vi "makeGraphLegend.vi"(7 "Front Panel Window:Minimum Size":T1, 10 "NewBnds":T2, 11 "XYGraph in":refnum<vi>) -> ()   [LabVIEW 2022 SP3]
uses:
  <vilib>/Utility/miscctls.llb/LVRectTypeDef.ctl
  <vilib>/Utility/miscctls.llb/LVPointTypeDef.ctl
  Anemometry/Anemometry Sub Vis/Data_plotting_vis/Results_plotter_Global.vi
panel:
  in  "Graph:Position:Left":i32=1
  in  "Graph:Position:Top":i32=26
  in  "baseLegendWidthChars":u32=33
  in  "origPlotAreaWidth":u32=510
  in  "origPlotAreaHeight":u32=256
  in  "avPixelsPerChar":dbl=6.0 format="%#_13g"
  in  "legendOffsetFromPlotArea":u32=117
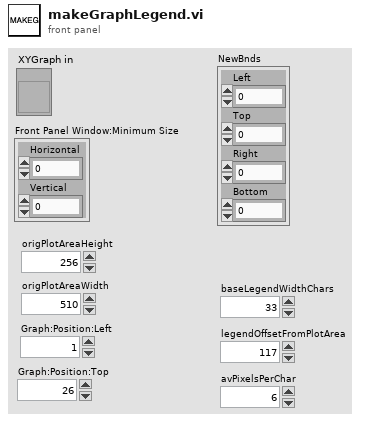
[diagram p1: front panel]
types:
  T1 = typedef "LVPointTypeDef.ctl" = cluster{"Horizontal":i16, "Vertical":i16}
  T2 = typedef "LVRectTypeDef.ctl" = cluster{"Left":i16, "Top":i16, "Right":i16, "Bottom":i16}
  T3 = cluster{"Plot Color":u32, "Plot Interpolation":u8, "Point Style":u8, "Line Style":u8, "Fill/Pt. Color":u32, "Line Width":u8, "Bar Plot Style":u8, "Fill To":i16}[]
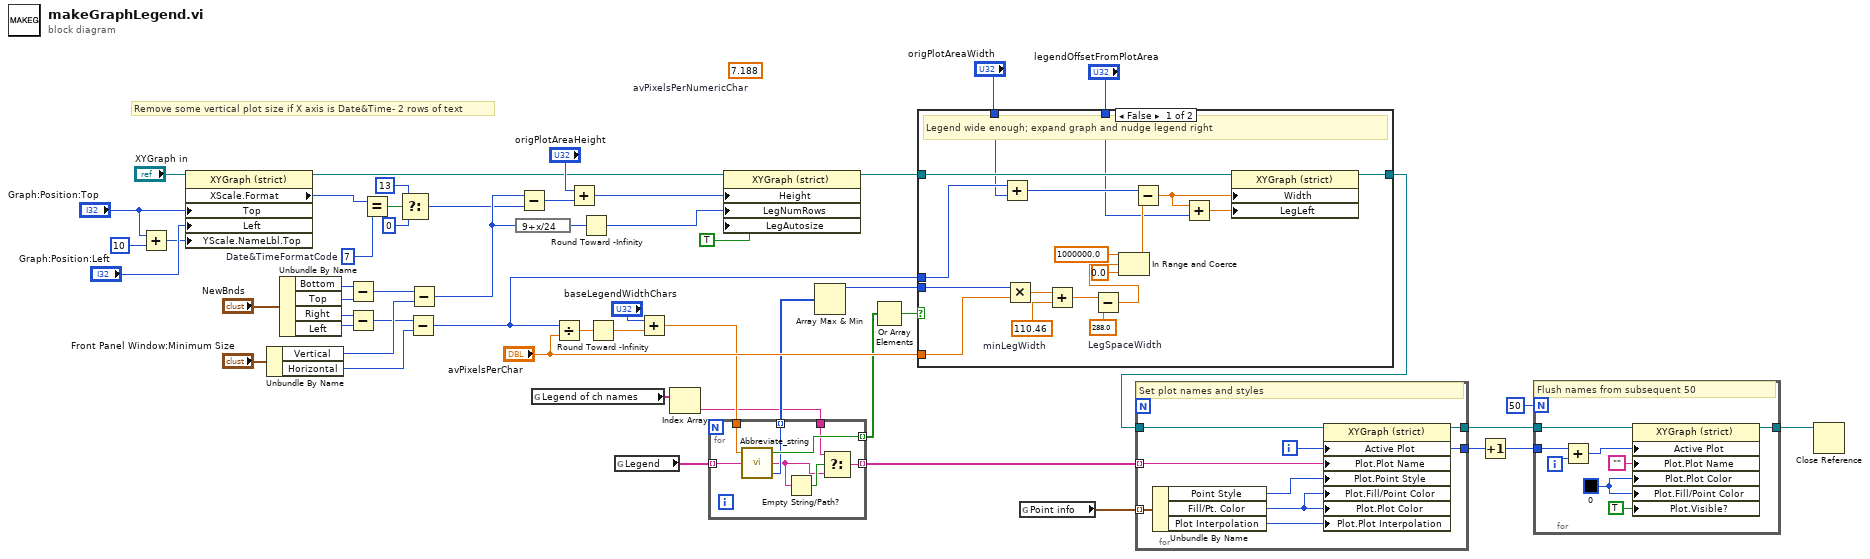
[diagram p0: block diagram]
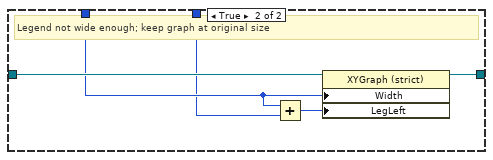
[diagram p2: hidden frame]
diagram:
  w12 = u8 7  # Date&TimeFormatCode
  (unwired) 7.188  # avPixelsPerNumericChar
  # "Remove some vertical plot size if X axis is Date&Time- 2 rows of text"
  n1 = Add(x="Graph:Position:Top", y=10) -> (x+y=w2:i32)
  n2 = property class="XYGraph (strict)"(reference="XYGraph in", "Top"="Graph:Position:Top", "Left"="Graph:Position:Left", "YScale.NameLbl.Top"=w2) -> (reference out=w14:refnum<vi>, "XScale.Format"=w13:u8)  [unwired: 1 in, 1 out]
  n3 = Unbundle By Name("Front Panel Window:Minimum Size") -> ("Vertical"=w43:i16, "Horizontal"=w34:i16)
  n4 = Unbundle By Name("NewBnds") -> ("Bottom"=w48:i16, "Top"=w49:i16, "Right"=w46:i16, "Left"=w45:i16)
  n5 = Subtract(x=w48, y=w49) -> (x-y=w50:i16)
  n6 = Subtract(x=w46, y=w45) -> (x-y=w35:i16)
  n7 = Equal?(x=w13, y=w12) -> (x = y?=w11:bool)
  n8 = Select(t=u8 13 ("y"), s=w11, f=u8 0) -> (s? t:f=w7:u8)
  n9 = Subtract(x=w35, y=w34) -> (x-y=w26:i16)
  n10 = Subtract(x=w50, y=w43) -> (x-y=w32:i16)
  n11 = expression code="9+x/24"(w32) -> (w39:i16)
  n12 = Subtract(x=w32, y=w7) -> (x-y=w8:i16)
  n13 = global read "Results_plotter_Global.vi" "Legend of ch names"() -> (w6:string[])
  n14 = Divide(x=w26, y="avPixelsPerChar") -> (x/y=w28:dbl)
  n15 = Add(x="origPlotAreaHeight", y=w8) -> (x+y=w31:u32)
  n16 = Round Toward -Infinity(1:w39) -> (0:w30:i16)
  n17 = Round Toward -Infinity(1:w28) -> (0:w27:dbl)
  n18 = global read "Results_plotter_Global.vi" "Legend"() -> (w53:string[])
  n19 = Add(x="baseLegendWidthChars", y=w27) -> (x+y=w24:dbl)
  n20 = Index Array(array=w6) -> (element=w5:string)  [unwired: 1 in]
  n21 = for {
    tunnel: w53 -> [w58] mode=indexing
    tunnel: w24 -> [w61]
    tunnel: [w54] -> w23 mode=indexing
    tunnel: [w60] -> w21 mode=indexing
    tunnel: [w59] -> w19 mode=indexing
    tunnel: w5 -> [w56]
    n22 = call "Abbreviate_string.vi"("Input String"=w58, "Max String Length"=w61) -> ("finalLength"=w59:i32, "Output String"=w55:string, "needMoreWidth"=w60:bool)  [unwired: 1 in]
    n23 = Empty String/Path?(string/path=w55) -> (empty?=w57:bool)
    n24 = Select(t=w56, s=w57, f=w55) -> (s? t:f=w54:string)
  }
  n25 = property on="Property Node" class="XYGraph (strict)"(reference=w14, "Height"=w31, "LegNumRows"=w30, "LegAutosize"=TRUE ("Legend:Autosize")) -> (reference out=w38:refnum<vi>)  [unwired: 1 in, 1 out]
  n26 = Array Max & Min(array=w19) -> (max value=w18:i32)  [unwired: 3 out]
  n27 = Or Array Elements(Boolean array=w21) -> (logical OR=w20:bool)
  n28 = case shown="False" w20 {
    tunnel: w38 -> [w78 w83]
    tunnel: [w79 w84] -> w36
    tunnel: w26 -> [w75 _]
    tunnel: w18 -> [w70 _]
    tunnel: "avPixelsPerChar" -> [w69 _]
    tunnel: "origPlotAreaWidth" -> [w63 w81]
    tunnel: "legendOffsetFromPlotArea" -> [w62 w80]
    frame False {
      w68 = 288.0  # LegSpaceWidth
      w71 = 110.46  # minLegWidth
      # "Legend wide enough; expand graph and nudge legend right"
      n29 = Add(x=w75, y=w63) -> (x+y=w74:u32)
      n30 = Multiply(x=w70, y=w69) -> (x*y=w72:dbl)
      n31 = Add(x=w72, y=w71) -> (x+y=w73:dbl)
      n32 = Subtract(x=w73, y=w68) -> (x-y=w66:dbl)
      n33 = In Range and Coerce(upper limit=1000000.0, x=w66, lower limit=0.0) -> (coerced(x)=w67:dbl)  [unwired: 1 out]
      n34 = Subtract(x=w74, y=w67) -> (x-y=w76:dbl)
      n35 = Add(x=w76, y=w62) -> (x+y=w77:dbl)
      n36 = property on="Property Node" class="XYGraph (strict)"(reference=w78, "Width"=w76, "LegLeft"=w77) -> (reference out=w79:refnum<vi>)  [unwired: 1 in, 1 out]
    }
    frame True {
      # "Legend not wide enough; keep graph at original size"
      n37 = Add(x=w81, y=w80) -> (x+y=w82:u32)
      n38 = property on="Property Node" class="XYGraph (strict)"(reference=w83, "Width"=w81, "LegLeft"=w82) -> (reference out=w84:refnum<vi>)  [unwired: 1 in, 1 out]
    }
  }
  n39 = global read "Results_plotter_Global.vi" "Point info"() -> (w52:T3)
  n40 = for {
    tunnel: w52 -> [w92] mode=indexing
    tunnel: w36 -> [w88]
    tunnel: [w87] -> w41
    tunnel: [w86] -> w42
    tunnel: w23 -> [w85] mode=indexing
    i -> [w86]
    # "Set plot names and styles"
    n41 = Unbundle By Name(w92) -> ("Point Style"=w91:u8, "Fill/Pt. Color"=w90:u32, "Plot Interpolation"=w89:u8)
    n42 = property on="Property Node" class="XYGraph (strict)"(reference=w88, "Active Plot"=w86, "Plot.Plot Name"=w85, "Plot.Point Style"=w91, "Plot.Fill/Point Color"=w90, "Plot.Plot Color"=w90, "Plot.Plot Interpolation"=w89) -> (reference out=w87:refnum<vi>)  [unwired: 1 in, 1 out]
  }
  n43 = Increment(x=w42) -> (x+1=w40:i32)
  n44 = for {
    N: 50 -> [_]
    tunnel: w41 -> [w98]
    tunnel: w40 -> [w94]
    tunnel: [w93] -> w22
    i -> [w100]
    w99 = u32 0
    # "Flush names from subsequent 50"
    n45 = Add(x=w94, y=w100) -> (x+y=w97:i32)
    n46 = property on="Property Node" class="XYGraph (strict)"(reference=w98, "Active Plot"=w97, "Plot.Plot Name"="", "Plot.Plot Color"=w99, "Plot.Fill/Point Color"=w99, "Plot.Visible?"=TRUE ("Plot.Visible")) -> (reference out=w93:refnum<vi>)  [unwired: 1 in, 1 out]
  }
  n47 = Close Reference(reference=w22) -> ()  [unwired: 1 in, 1 out]
